vi "Save_to_Project.vi"(6 "commonPath":path, 8 "error in (no error)":errorcluster, 9 "index":i32, 10 "buildObject":T1, 11 "AB_Destination in":refnum<class "AB_Destination.lvclass">) -> (0 "error out":errorcluster, 3 "AB_Destination out":refnum<class "AB_Destination.lvclass">)   [LabVIEW 2020, in "AB_Destination.lvclass"]
uses:
  <vilib>/AppBuilder/AB_Classes/Destination/AB_Destination.lvclass
  <resource>/Framework/Providers/API/ItemRef.ctl
  <vilib>/AppBuilder/AB_Classes/Destination/AB_Destination.lvclass/AB_Destination.ctl
  <vilib>/AppBuilder/RW_Project/AB_RW_Project_Destination_Data.ctl
  <vilib>/AppBuilder/RW_Project/AB_RW_Project_PropBag_Action.ctl
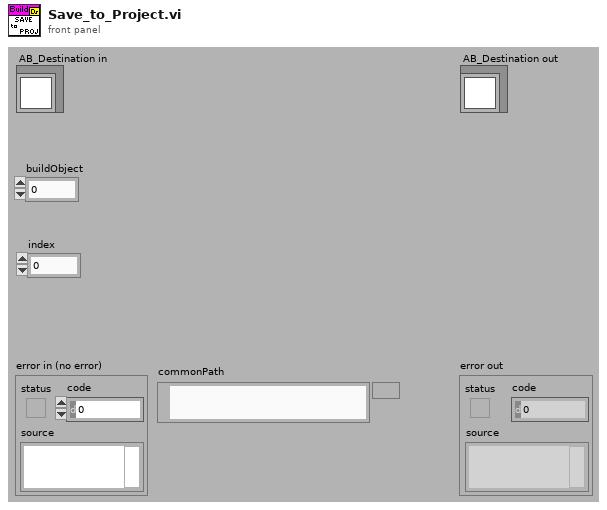
[diagram p1: front panel]
types:
  T1 = typedef "ItemRef.ctl" = u64
  T2 = typedef "AB_RW_Project_Destination_Data.ctl" = cluster{"destName":string, "path":path, "preserveHierarchy":bool, "libraryName":string}
  T3 = typedef "AB_RW_Project_PropBag_Action.ctl" = enum16{"read", "write", "clear", "readPrevious", "writePrevious", "clearPrevious"}
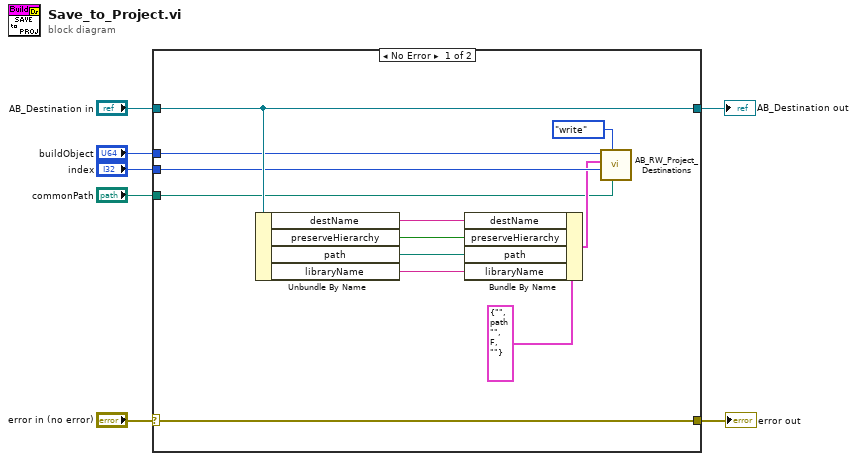
[diagram p0: block diagram]
diagram:
  n1 = case shown="No Error" "error in (no error)" {
    selector: "error in (no error)" -> [w19 w21]
    tunnel: [w19 w21] -> w6
    tunnel: [w18 w20] -> w4
    tunnel: "AB_Destination in" -> [w18 w20]
    tunnel: "index" -> [w17 _]
    tunnel: "buildObject" -> [w14 _]
    tunnel: "commonPath" -> [w10 _]
    frame No Error {
      n2 = Unbundle By Name(w18) -> ("destName"=w12:string, "preserveHierarchy"=w11:bool, "path"=w9:path, "libraryName"=w8:string)
      n3 = Bundle By Name(cluster=T2 {"destName"="", "path"=path "", "preserveHierarchy"=FALSE, "libraryName"=""} ("data in"), "destName"=w12, "preserveHierarchy"=w11, "path"=w9, "libraryName"=w8) -> (w15:T2)
      n4 = call <vilib>:"AB_RW_Project_Destinations.vi"("ProjectPath"=w10, "action"=AB_RW_Project_PropBag_Action."write", "index"=w17, "data in"=w15, "buildObject"=w14) -> ()  [unwired: 1 in, 6 out]
    }
    frame Error {
    }
  }
  "error out" <- w6
  "AB_Destination out" <- w4
